vi "Jedanmotor.vi"() -> ()   [LabVIEW 2014]
uses:
  <vilib>/rvi/Emulation/niFpgaGetClockAttributes.vi
  <vilib>/rvi/Emulation/niFpgaSctlEmulationGetInTimedLoop.vi
  <vilib>/rvi/Emulation/niFpgaEmulationReportErrorSimple.vi
  <vilib>/rvi/eio/common/nirviEmuTemplateMethod_errors.vi
  <vilib>/rvi/Emulation/niFpgaCriticalErrorInLSC.vi
  <vilib>/eio/EIONode/EIONode.xnode
panel:
  in  "smjer":bool
  in  "korak/polukorak":bool
  in  "stop":bool
  in  "step":sgl(knob) scale=0.0..300.0
  in  "enable":bool
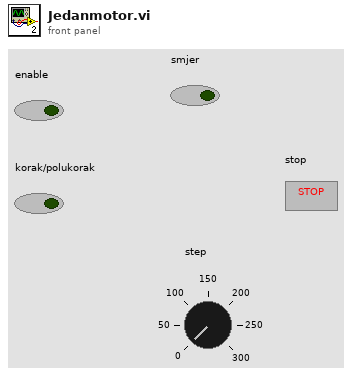
[diagram p1: front panel]
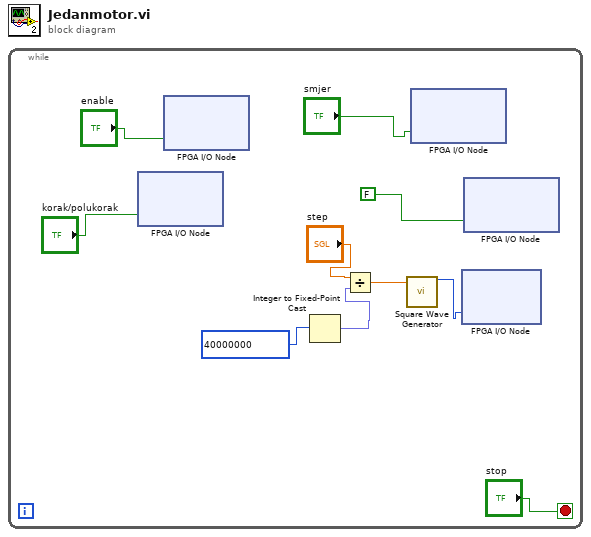
[diagram p0: block diagram]
diagram:
  n1 = while {
    stop <- "stop" stop-if-true
    n2 = xnode "FPGA I/O Node"("DIO7"="korak/polukorak") -> ()  [unwired: 1 in, 1 out]
    n3 = xnode "FPGA I/O Node"("DIO4"="enable") -> ()  [unwired: 1 in, 1 out]
    n4 = Integer to Fixed-Point Cast(integer=40000000) -> (fixed-point=w8:fxp<+/-,32,32>)  [unwired: 1 in]
    n5 = Divide(x="step", y=w8) -> (x/y=w7:sgl)
    n6 = call "Square Wave Generator"("frequency (periods/tick)"=w7) -> ("square wave out"=w6:i16)  [unwired: 14 in]
    n7 = xnode "FPGA I/O Node"("DIO13"="smjer") -> ()  [unwired: 1 in, 1 out]
    n8 = xnode "FPGA I/O Node"("AO1"=w6) -> ()  [unwired: 1 in, 1 out]
    n9 = xnode "FPGA I/O Node"("DIO10"=FALSE) -> ()  [unwired: 1 in, 1 out]
  }
